vi "AB_820_850_Project_EXE_Info.vi"(7 "action":T1, 8 "error in (no error)":errorcluster, 10 "Exe_info in":T2, 11 "Object In":T3) -> (0 "error out":errorcluster, 2 "Exe info out":T2, 3 "Object Out":T3)   [LabVIEW 2020]
uses:
  <resource>/Framework/Providers/API/ItemRef.ctl
  <vilib>/AppBuilder/RW_Project/AB_RW_Project_PropBag_Action.ctl
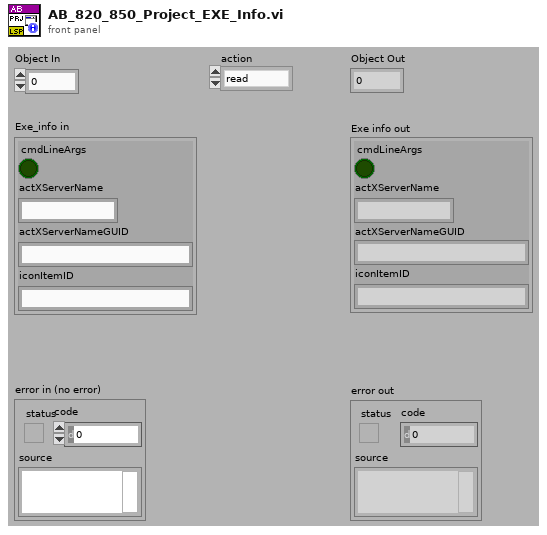
[diagram p1: front panel]
types:
  T1 = typedef "AB_RW_Project_PropBag_Action.ctl" = enum16{"read", "write", "clear", "readPrevious", "writePrevious", "clearPrevious"}
  T2 = cluster{"cmdLineArgs":bool, "actXServerName":string, "actXServerNameGUID":string, "iconItemID":string}
  T3 = typedef "ItemRef.ctl" = u64
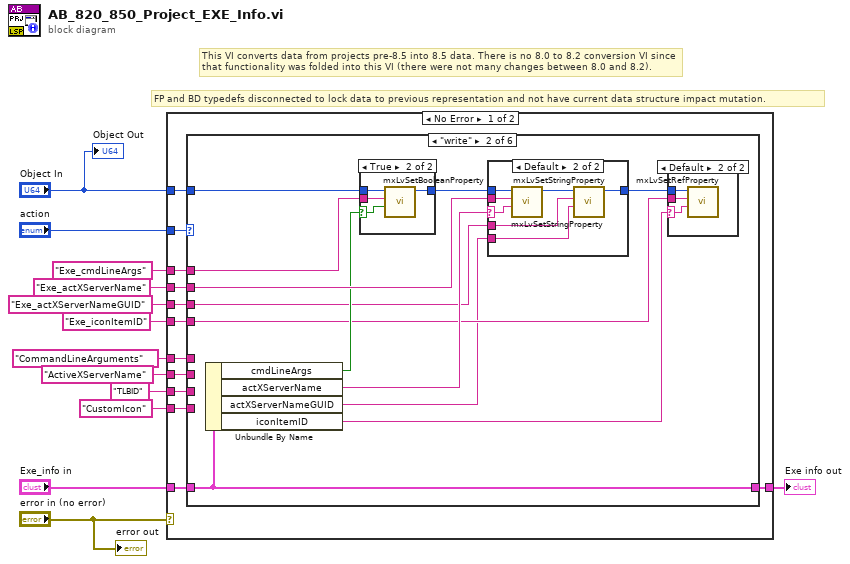
[diagram p0: block diagram]
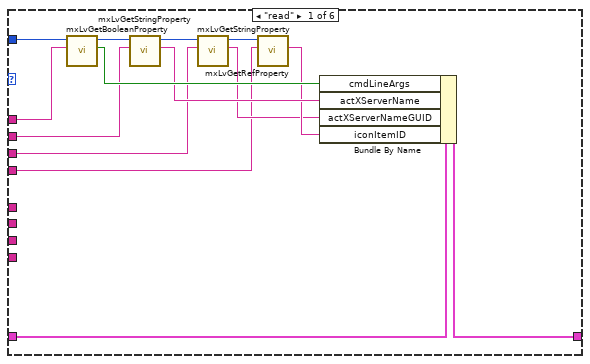
[diagram p2: hidden frame]
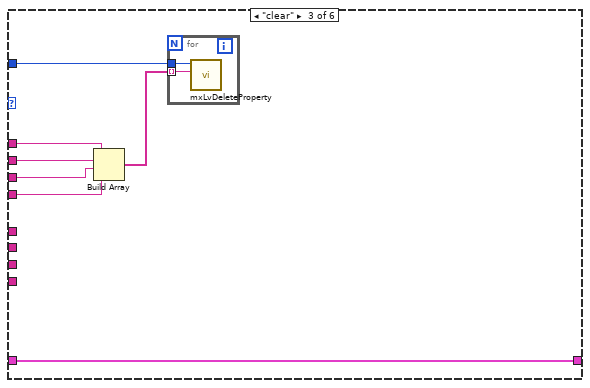
[diagram p6: hidden frame]
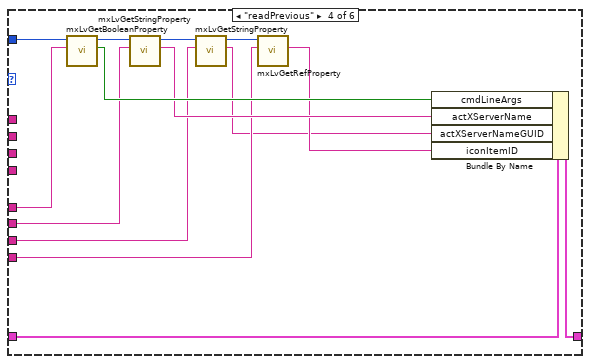
[diagram p7: hidden frame]
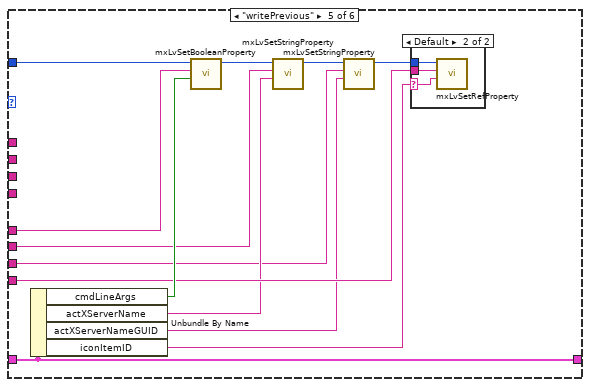
[diagram p8: hidden frame]
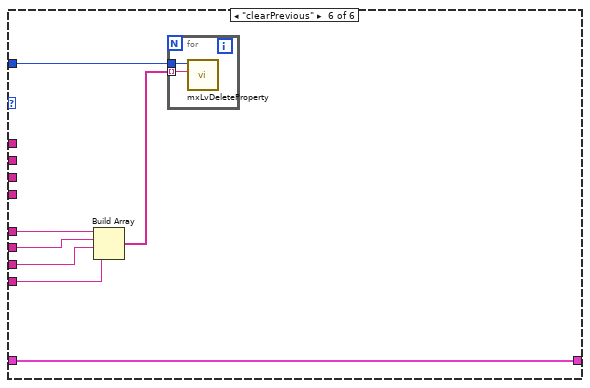
[diagram p10: hidden frame]
diagram:
  # "FP and BD typedefs disconnected to lock data to previous representation and not have current data structure impact mutation."
  # "This VI converts data from projects pre-8.5 into 8.5 data. There is no 8.0 to 8.2 conversion VI since that functionality was folded into this VI (there were not many changes between 8.0 and 8.2)."
  n1 = case shown="No Error" "error in (no error)" {
    tunnel: "Object In" -> [w23 _]
    tunnel: [w25 _] -> w11
    tunnel: "Exe_cmdLineArgs" -> [w24 _]
    tunnel: "Exe_actXServerName" -> [w22 _]
    tunnel: "Exe_actXServerNameGUID" -> [w21 _]
    tunnel: "Exe_info in" -> [w20 _]
    tunnel: "action" -> [w19 _]
    tunnel: "CommandLineArguments" -> [w18 _]
    tunnel: "ActiveXServerName" -> [w17 _]
    tunnel: "CustomIcon" -> [w16 _]
    tunnel: "Exe_iconItemID" -> [w15 _]
    tunnel: "TLBID" -> [w14 _]
    frame No Error {
      n2 = case shown="\"write\"" w19 {
        tunnel: [w35 w47 w74 w86 w101 w113] -> w25
        tunnel: w24 -> [w34 w46 w71 _ _ _]
        tunnel: w23 -> [w33 w51 w73 w85 w103 w112]
        tunnel: w22 -> [w32 w48 w72 _ _ _]
        tunnel: w21 -> [w28 w40 w70 _ _ _]
        tunnel: w20 -> [w31 w47 w74 w84 w101 w113]
        tunnel: w18 -> [_ _ _ w83 w98 w109]
        tunnel: w17 -> [_ _ _ w82 w97 w110]
        tunnel: w16 -> [_ _ _ w81 w96 w108]
        tunnel: w15 -> [w26 w42 w68 _ _ _]
        tunnel: w14 -> [_ _ _ w78 w91 w107]
        frame "read" {
          n3 = call <resource>:"mxLvGetBooleanProperty.vi"("Tag"=w34, "Item"=w33) -> ("Value"=w38:bool, "Item"=w39:T3)  [unwired: 7 in, 1 out]
          n4 = call <resource>:"mxLvGetStringProperty.vi"("Tag"=w32, "Item"=w39) -> ("Value"=w37:string, "Item"=w30:T3)  [unwired: 7 in, 1 out]
          n5 = call <resource>:"mxLvGetStringProperty.vi"("Tag"=w28, "Item"=w30) -> ("Value"=w27:string, "Item"=w29:T3)  [unwired: 7 in, 1 out]
          n6 = call <resource>:"mxLvGetRefProperty.vi"("Tag"=w26, "Item"=w29) -> ("Value"=w36:string)  [unwired: 7 in, 2 out]
          n7 = Bundle By Name(cluster=w31, "cmdLineArgs"=w38, "actXServerName"=w37, "actXServerNameGUID"=w27, "iconItemID"=w36) -> (w35:T2)
        }
        frame "write" {
          n8 = Unbundle By Name(w47) -> ("cmdLineArgs"=w45:bool, "actXServerName"=w44:string, "actXServerNameGUID"=w41:string, "iconItemID"=w43:string)
          n9 = case shown="True" w45 {
            selector: w45 -> [_ w64]
            tunnel: w51 -> [w63 w67]
            tunnel: [w63 w66] -> w50
            tunnel: w46 -> [_ w65]
            frame False {
            }
            frame True {
              n10 = call <resource>:"mxLvSetBooleanProperty.vi"("Value (F)"=w64, "Tag"=w65, "Item"=w67) -> ("Item"=w66:T3)  [unwired: 7 in, 1 out]
            }
          }
          n11 = case shown="Default" w44 {
            selector: w44 -> [_ w60]
            tunnel: w50 -> [w55 w62]
            tunnel: [w55 w58] -> w49
            tunnel: w48 -> [_ w61]
            tunnel: w41 -> [_ w57]
            tunnel: w40 -> [_ w56]
            frame "" {
            }
            frame Default {
              n12 = call <resource>:"mxLvSetStringProperty.vi"("Value (\"\")"=w60, "Tag"=w61, "Item"=w62) -> ("Item"=w59:T3)  [unwired: 7 in, 1 out]
              n13 = call <resource>:"mxLvSetStringProperty.vi"("Value (\"\")"=w57, "Tag"=w56, "Item"=w59) -> ("Item"=w58:T3)  [unwired: 7 in, 1 out]
            }
          }
          n14 = case shown="Default" w43 {
            selector: w43 -> [_ w52]
            tunnel: w49 -> [_ w54]
            tunnel: w42 -> [_ w53]
            frame "" {
            }
            frame Default {
              n15 = call <resource>:"mxLvSetRefProperty.vi"("Value (\"\")"=w52, "Tag"=w53, "Item"=w54) -> ()  [unwired: 7 in, 2 out]
            }
          }
        }
        frame "clear" {
          n16 = Build Array(w71, w72, w70, w68) -> (w69:string[])
          n17 = for {
            tunnel: w73 -> [w76]
            tunnel: w69 -> [w75] mode=indexing
            n18 = call <resource>:"mxLvDeleteProperty.vi"("Tag"=w75, "Item"=w76) -> ()  [unwired: 8 in, 2 out]
          }
        }
        frame "readPrevious" {
          n19 = call <resource>:"mxLvGetBooleanProperty.vi"("Tag"=w83, "Item"=w85) -> ("Value"=w89:bool, "Item"=w90:T3)  [unwired: 7 in, 1 out]
          n20 = call <resource>:"mxLvGetStringProperty.vi"("Tag"=w82, "Item"=w90) -> ("Value"=w88:string, "Item"=w80:T3)  [unwired: 7 in, 1 out]
          n21 = call <resource>:"mxLvGetStringProperty.vi"("Tag"=w78, "Item"=w80) -> ("Value"=w77:string, "Item"=w79:T3)  [unwired: 7 in, 1 out]
          n22 = call <resource>:"mxLvGetRefProperty.vi"("Tag"=w81, "Item"=w79) -> ("Value"=w87:string)  [unwired: 7 in, 2 out]
          n23 = Bundle By Name(cluster=w84, "cmdLineArgs"=w89, "actXServerName"=w88, "actXServerNameGUID"=w77, "iconItemID"=w87) -> (w86:T2)
        }
        frame "writePrevious" {
          n24 = Unbundle By Name(w101) -> ("cmdLineArgs"=w100:bool, "actXServerName"=w95:string, "actXServerNameGUID"=w92:string, "iconItemID"=w99:string)
          n25 = call <resource>:"mxLvSetBooleanProperty.vi"("Value (F)"=w100, "Tag"=w98, "Item"=w103) -> ("Item"=w102:T3)  [unwired: 7 in, 1 out]
          n26 = call <resource>:"mxLvSetStringProperty.vi"("Value (\"\")"=w95, "Tag"=w97, "Item"=w102) -> ("Item"=w94:T3)  [unwired: 7 in, 1 out]
          n27 = call <resource>:"mxLvSetStringProperty.vi"("Value (\"\")"=w92, "Tag"=w91, "Item"=w94) -> ("Item"=w93:T3)  [unwired: 7 in, 1 out]
          n28 = case shown="Default" w99 {
            selector: w99 -> [_ w104]
            tunnel: w93 -> [_ w106]
            tunnel: w96 -> [_ w105]
            frame "" {
            }
            frame Default {
              n29 = call <resource>:"mxLvSetRefProperty.vi"("Value (\"\")"=w104, "Tag"=w105, "Item"=w106) -> ()  [unwired: 7 in, 2 out]
            }
          }
        }
        frame "clearPrevious" {
          n30 = Build Array(w109, w110, w107, w108) -> (w111:string[])
          n31 = for {
            tunnel: w112 -> [w115]
            tunnel: w111 -> [w114] mode=indexing
            n32 = call <resource>:"mxLvDeleteProperty.vi"("Tag"=w114, "Item"=w115) -> ()  [unwired: 8 in, 2 out]
          }
        }
      }
    }
    frame Error {
    }
  }
  "Exe info out" <- w11
  "Object Out" <- "Object In"
  "error out" <- "error in (no error)"
